vi "FRCts20_WebMethods_Events_GET.vi"(7 "httpRequestID":u32, 11 "view":string) -> ()   [LabVIEW 2013, in "FRCts20_WebMethods.lvlib"]
doc: "<B>GET</B> on the specified <B>competition</B> resource\n\n<B>Default Return:</B> <B>competition</B> information and list of contained divisions\n\n<B>query =</B> info - Returns only <B>competition</B> information\n stats - Returns statistics for <B>competition</B>\n images - Returns .png and .jpeg images for <B>competition</B>\n videos - Returns .wmv videos for <B>competition</B>\n\nhttp://<server address>:<port>/FRCts/competition/<B>competition</B>"
uses:
  FRCts20_WebMethods.lvlib
  Backend/source/VI Source/FRCts20_Backend_API/FRCts20_Backend_API.lvlib
  <vilib>/wsapi/NI_WebServices.lvlib
  ESP Engine/source/VI Source/FRCts20_EspEngine.lvlib
  Backend/source/VI Source/FRCts20_Backend_API/FRCts20_Backend_API_Command_EventRoot.ctl
  Backend/source/VI Source/FRCts20_Backend_API/FRCts20_Backend_API_EventRoot.vi
panel:
  out "error out":errorcluster
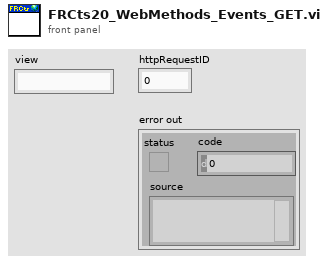
[diagram p1: front panel]
types:
  T1 = typedef "FRCts20_Backend_API.lvlib/FRCts20_Backend_API_Command_EventRoot.ctl" = string
  T2 = typedef "FRCts20_EspEngine.lvlib/FRCts20_EspEngine_SearchBrowser.ctl" = cluster{"Event":cluster{"Event Index":u32, "Event Name":string, "Start Time":timestamp, "End Time":timestamp, "OpenIssues":u8, "IsLive":bool}[], "select-choice-software":string, "select-choice-location":string}
  T3 = typedef "FRCts20_Backend_API.lvlib/FRCts20_Backend_API_EventRoot.ctl" = cluster{"Event":cluster{"Event Index":u32, "Event Name":string, "Start Time":timestamp, "End Time":timestamp, "OpenIssues":u8, "IsLive":bool}[], "APIReturn":string}
  T4 = typedef "FRCts20_WebMethods.lvlib/FRCts20_WebMethods_ctl_returntype.ctl" = string
  T5 = typedef "FRCts20_EspEngine.lvlib/FRCts20_EspEngine_Universe.ctl" = cluster{"TeamsListLength":i16, "Teams":T6[], "LiveEventListLength":i16, "LiveEvents":T12[], "NonLiveEventListLength":i16, "NonLiveEvents":T12[], "OpenIssueCount":i16, "NotFoundStatus":bool}
  T6 = typedef "FRCts20_EspEngine.lvlib/FRCts20_EspEngine_Team.ctl" = cluster{"Team":T7, "RequestListLength":i16, "Requests":T10[]}
  T7 = typedef "FRCts20_WebMethods.lvlib/FRCts20_WebMethods_ctl_singleTeam.ctl" = cluster{"Events":string[], "Robot Name":string, "Kinect":bool, "Vision":bool, "Can":bool, "Tags":string, "Avatar URL":string, "Team":T8, "SWType":T9}
  T8 = typedef "FRCts20_WebMethods.lvlib/FRCts20_WebMethods_ctl_teamIdentifier.ctl" = cluster{"Team Nickname":string, "Team Number ":u32, "UniqueId":u32}
  T9 = typedef "FRCts20_Backend_API.lvlib/FRCts20_Backend_API_SW.ctl" = string
  T10 = typedef "FRCts20_WebMethods.lvlib/FRCts20_WebMethods_ctl_request.ctl" = cluster{"Event":string, "Description":string, "Status":T11, "Open Date":string, "Last Update":string, "Close Date":string, "UniqueId":i32, "Team":cluster{"Team Nickname":string, "Team Number ":i32, "UniqueId":i32}, "Comments":cluster{"Request Number":dbl, "Text":string, "Author":string, "IsSolution":bool, "Team":cluster{"Team Nickname":string, "Team Identifier ":dbl}, "UniqueId":i32}[]}
  T11 = typedef "FRCts20_Backend_API.lvlib/FRCts20_Backend_API_Status.ctl" = enum16{"Open", "In Work", "Closed"}
  T12 = typedef "FRCts20_EspEngine.lvlib/FRCts20_EspEngine_Event.ctl" = cluster{"Single Event":T13, "EventOpenIssueCount":i16, "Requests":cluster{"RequestId":i32, "Request Description":string, "Team Number":i32}[], "ClosedRequests":cluster{"RequestId":i32, "Request Description":string, "Team Number":i32}[], "NotFoundStatus":bool}
  T13 = typedef "FRCts20_WebMethods.lvlib/FRCts20_WebMethods_ctl_singleEvent.ctl" = cluster{"Team":T8[], "Issue Count":i32, "Location":string, "Start Date ":timestamp}
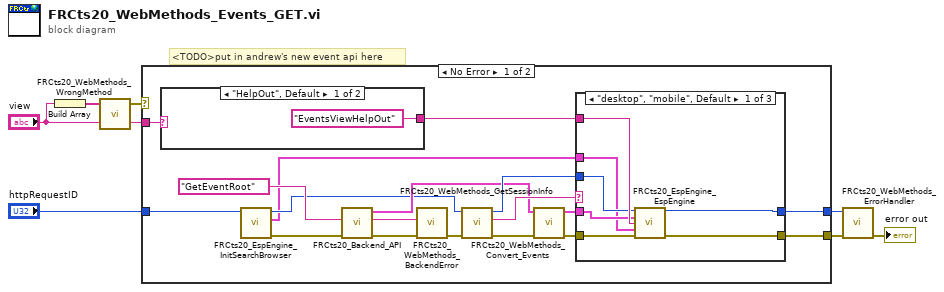
[diagram p0: block diagram]
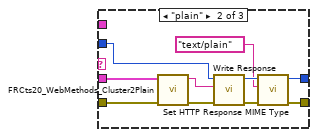
[diagram p2: hidden frame]
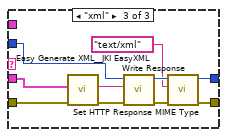
[diagram p3: hidden frame]
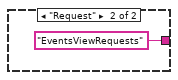
[diagram p4: hidden frame]
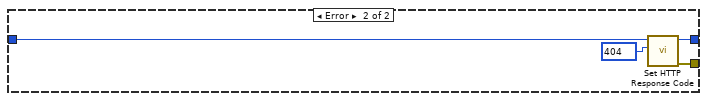
[diagram p5: hidden frame]
diagram:
  # "<TODO>put in andrew's new event api here"
  n1 = Build Array("view") -> (w2:string[])
  n2 = call "FRCts20_WebMethods_WrongMethod.vi"("Method Inputs"=w2) -> ("error out"=w1:errorcluster)  [unwired: 4 in]
  n3 = case shown="No Error" w1 {
    tunnel: "httpRequestID" -> [w11 w58]
    tunnel: [w21 w56] -> w6
    tunnel: [w20 w57] -> w5
    tunnel: "view" -> [w25 _]
    frame No Error {
      n4 = case shown="\"HelpOut\", Default" w25 {
        tunnel: ["EventsViewHelpOut" "EventsViewRequests"] -> w15
        frame "HelpOut", Default {
        }
        frame "Request" {
        }
      }
      n5 = call "FRCts20_EspEngine_InitSearchBrowser.vi"("httpRequestID"=w11) -> ("error out"=w9:errorcluster, "SearchBrowser"=w8:T2, "httpRequestID out"=w10:u32)  [unwired: 8 in]
      n6 = call-poly "FRCts20_Backend_API.vi"("error in (no error)"=w9, "Message"=T1 "GetEventRoot") -> ("error out"=w16:errorcluster, "Status"=w19:string, "EventRoot Out"=w17:T3)  [unwired: 7 in]
      n7 = call "FRCts20_WebMethods_BackendError.vi"("error in (no error)"=w16, "Status"=w19) -> ("error out"=w22:errorcluster)  [unwired: 8 in, 1 out]
      n8 = call "FRCts20_WebMethods_GetSessionInfo.vi"("error in"=w22, "httpRequestID"=w10) -> ("error out"=w13:errorcluster, "Return Type"=w24:T4, "httpRequestID out"=w23:u32)  [unwired: 7 in]
      n9 = call "FRCts20_WebMethods_Convert_Events.vi"("error in (no error)"=w13, "EventRoot Out"=w17) -> ("error out"=w12:errorcluster, "Universe"=w14:T5)  [unwired: 8 in]
      n10 = case shown="\"desktop\", \"mobile\", Default" w24 {
        tunnel: w23 -> [w29 w42 w52]
        tunnel: [w30 w39 w46] -> w20
        tunnel: [w31 w38 w47] -> w21
        tunnel: w15 -> [w32 _ _]
        tunnel: w14 -> [w27 w34 w44]
        tunnel: w12 -> [w28 w33 w43]
        tunnel: w8 -> [w26 _ _]
        frame "desktop", "mobile", Default {
          n11 = call "FRCts20_EspEngine_EspEngine.vi"("httpRequestID"=w29, "Cluster"=w27, "Page"=w32, "SearchBrowser"=w26, "error in (no error)"=w28) -> ("httpRequestID out"=w30:u32, "error out"=w31:errorcluster)  [unwired: 9 in]
        }
        frame "plain" {
          n12 = call "FRCts20_WebMethods_Cluster2Plain.vi"("error in (no error)"=w33, "Cluster"=w34) -> ("error out"=w37:errorcluster, "plain text"=w36:string)  [unwired: 8 in]
          n13 = call <vilib>:"Write Response.vi"("error in (no error)"=w37, "response string"=w36, "httpRequestID"=w42) -> ("error out"=w41:errorcluster, "httpRequestID out"=w40:u32)  [unwired: 7 in]
          n14 = call <vilib>:"Set HTTP Response MIME Type.vi"("error in (no error)"=w41, "MIME type (text/html)"="text/plain", "httpRequestID"=w40) -> ("error out"=w38:errorcluster, "httpRequestID out"=w39:u32)  [unwired: 7 in]
        }
        frame "xml" {
          n15 = call <vilib>:"Easy Generate XML__JKI EasyXML.vi"("error in (no error)"=w43, "LabVIEW Data"=w44) -> ("error out"=w51:errorcluster, "XML String"=w50:string)  [unwired: 8 in]
          n16 = call <vilib>:"Write Response.vi"("error in (no error)"=w51, "response string"=w50, "httpRequestID"=w52) -> ("error out"=w48:errorcluster, "httpRequestID out"=w49:u32)  [unwired: 7 in]
          n17 = call <vilib>:"Set HTTP Response MIME Type.vi"("error in (no error)"=w48, "MIME type (text/html)"="text/xml", "httpRequestID"=w49) -> ("error out"=w47:errorcluster, "httpRequestID out"=w46:u32)  [unwired: 7 in]
        }
      }
    }
    frame Error {
      w55 = 404 items=["100"=100, "101"=101, "200"=200, "201"=201, "202"=202, "203"=203, "204"=204, "205"=205, "206"=206, "300"=300, "301"=301, "302"=302, "303"=303, "304"=304, "305"=305, "306"=306, "307"=307, "400"=400, "401"=401, "402"=402, "403"=403, "404"=404, "405"=405, "406"=406, "407"=407, "408"=408, "409"=409, "410"=410, "411"=411, "412"=412, "413"=413, "414"=414, "415"=415, "416"=416, "417"=417, "500"=500, "501"=501, "502"=502, "503"=503, "504"=504, "505"=505] ("response code (200)")
      n18 = call <vilib>:"Set HTTP Response Code.vi"("response code (200)"=w55, "httpRequestID"=w58) -> ("error out"=w56:errorcluster, "httpRequestID out"=w57:u32)  [unwired: 8 in]
    }
  }
  n19 = call "FRCts20_WebMethods_ErrorHandler.vi"("error in"=w6, "httpRequestID"=w5) -> ("error out"=→"error out":errorcluster)  [unwired: 9 in]
